vi "Ciclo for.vi"() -> ()   [LabVIEW 2016]
panel:
  out "Shift Register":dbl
  out "Last Value":dbl
  out "Array 2":dbl[](array[numeric])
  in  "N":i32
  out "Array":dbl[](array[numeric])
  out "Fibonacci":dbl
  out "Numeric":i32
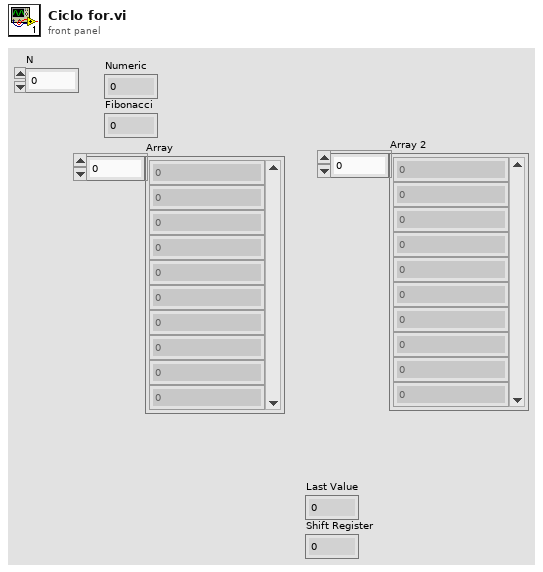
[diagram p1: front panel]
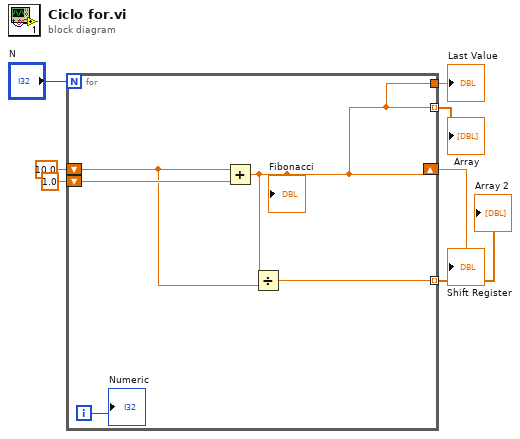
[diagram p0: block diagram]
diagram:
  n1 = for {
    N: "N" -> [_]
    shift-right: [w8] -> w1
    shift-left: 10.0 -> [w10]
    shift-left: 1.0 -> [w11]
    tunnel: [w8] -> w5 mode=indexing
    tunnel: [w9] -> w3 mode=indexing
    tunnel: [w8] -> w2
    i -> [w12]
    n2 = Add(x=w10, y=w11) -> (x+y=w8:dbl)
    "Fibonacci" <- w8
    n3 = Divide(x=w8, y=w10) -> (x/y=w9:dbl)
    "Numeric" <- w12
  }
  "Array" <- w5
  "Array 2" <- w3
  "Last Value" <- w2
  "Shift Register" <- w1
